vi "19052 PreSet_STEP_HOLD_time.vi"(8 "error in (no error)":errorcluster, 9 "string in":string, 11 "VISA resource in":refnum<visa-resource-name>) -> (0 "error out":errorcluster, 2 "output command":string, 3 "VISA resource out":refnum<visa-resource-name>)   [LabVIEW 2015]
doc: "This VI writes to the instrument the STEP HOLD time."
panel:
  # "PreSet STEP HOLD time"
  # "[sec]"
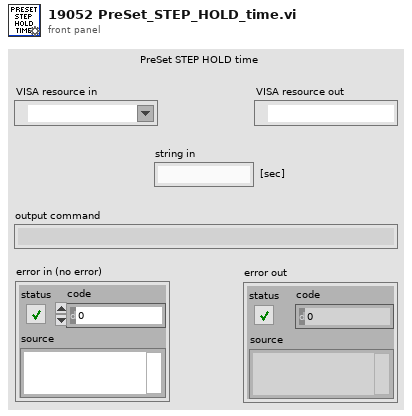
[diagram p1: front panel]
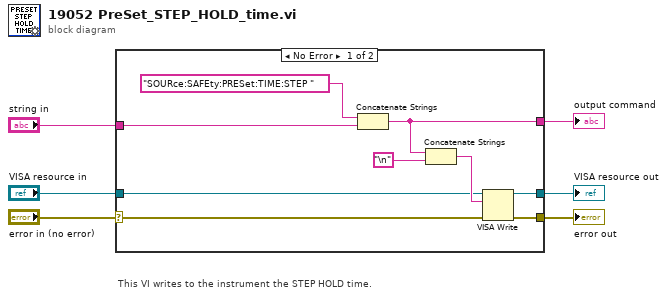
[diagram p0: block diagram]
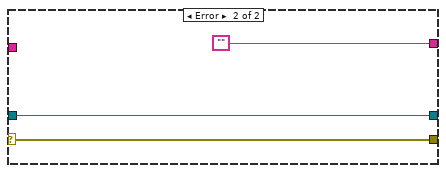
[diagram p2: hidden frame]
diagram:
  # "This VI writes to the instrument the STEP HOLD time."
  n1 = case shown="No Error" "error in (no error)" {
    selector: "error in (no error)" -> [w14 w18]
    tunnel: [w15 w18] -> w6
    tunnel: [w10 w17] -> w4
    tunnel: [w9 ""] -> w3
    tunnel: "string in" -> [w8 _]
    tunnel: "VISA resource in" -> [w7 w17]
    frame No Error {
      n2 = Concatenate Strings("SOURce:SAFEty:PRESet:TIME:STEP ", w8) -> (w9:string)
      n3 = Concatenate Strings(w9, "\n") -> (w12:string)
      n4 = VISA Write(VISA resource name=w7, write buffer=w12, error in (no error)=w14) -> (VISA resource name out=w10:refnum<visa-resource-name>, error out=w15:errorcluster)  [unwired: 1 out]
    }
    frame Error {
    }
  }
  "error out" <- w6
  "VISA resource out" <- w4
  "output command" <- w3
